vi "ExSubCloseMultStrip.vi"(1 "error in (no error)":errorcluster, 2 "Handles In":T1) -> (0 "error out":errorcluster)   [LabVIEW 2010]
panel:
  # "ExSubCloseMult:\nThis sub vi closes the multiple camera experiment."
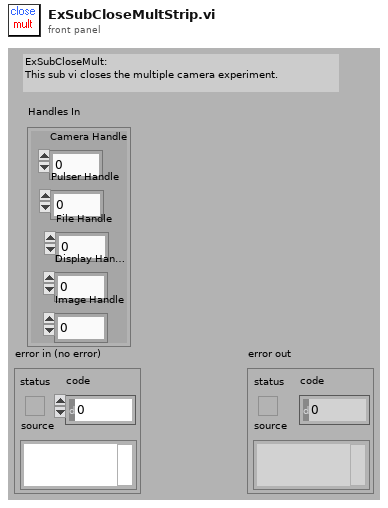
[diagram p1: front panel]
types:
  T1 = cluster{"Camera Handle":u32, "Pulser Handle":u32, "File Handle":u32, "Display Handle":u32, "Image Handle":u32}
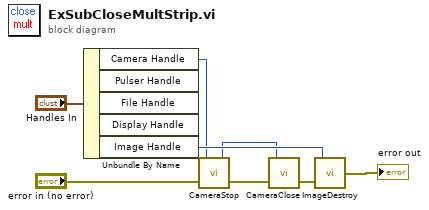
[diagram p0: block diagram]
diagram:
  n1 = Unbundle By Name("Handles In") -> ("Camera Handle"=w3:u32, "Image Handle"=w7:u32)  [unwired: 3 out]
  n2 = call <userlib>:"CameraStop.vi"("error in"="error in (no error)", "Camera Handle"=w3) -> ("error out"=w1:errorcluster, "Camera Handle"=w6:u32)
  n3 = call <userlib>:"CameraClose.vi"("error in"=w1, "Camera Handle"=w6) -> ("error out"=w4:errorcluster)
  n4 = call <userlib>:"ImageDestroy.vi"("error in"=w4, "Data handle"=w7) -> ("error out"=→"error out":errorcluster)
